vi "HFRR ADV v07.vi"() -> ()   [LabVIEW 2025] (continued)
                    n2291 = local write "Start Time"(TRUE ("Start Time")) -> ()
                    n2292 = property on="Stroke 2" class="DigNum (strict)"("Visible"=FALSE) -> ()  [unwired: 2 in, 2 out]
                    n2293 = case shown="False" w2888 {
                      frame False {
                        n2294 = property on="Heater Button" class="Bool (strict)"("DisabledEnum"=T15."Enabled" ("Disabled")) -> ()  [unwired: 2 in, 2 out]
                        n2295 = property on="Humidity" class="Bool (strict)"("DisabledEnum"=T15."Enabled" ("Disabled")) -> ()  [unwired: 2 in, 2 out]
                      }
                      frame True {
                      }
                    }
                    n2296 = case shown="False" "TestCompFlg" {
                      frame False {
                        n2297 = local read "StartFlg"() -> (w2896:bool)
                        n2298 = case shown="True" w2896 {
                          frame False {
                          }
                          frame True {
                            n2299 = flat-sequence {
                              frame #0 {
                                n2300 = local read "EVENT LOG"() -> (w2898:string)
                                n2301 = call "Event Log.vi"("Content"="Test was interrupted", "EVENT LOG"=w2898) -> ("EVENT LOG"=w2899:string)  [unwired: 8 in, 1 out]
                                n2302 = local write "EVENT LOG"(w2899) -> ()
                              }
                              frame #1 {
                                w2900 = FALSE ("StartFlg")
                                n2303 = local write "Heater Button"(w2900) -> ()
                                n2304 = local write "StartFlg"(w2900) -> ()
                                n2305 = local write "Humidity"(w2900) -> ()
                              }
                            }
                          }
                        }
                      }
                      frame True {
                      }
                    }
                    n2306 = local write "String 14"("Test will autostart once parameters reach the set value." ("String 14")) -> ()
                  }
                  frame True {
                    (unwired) FALSE ("Visible")
                    n2307 = property on="Stroke 2" class="DigNum (strict)"("Visible"=TRUE) -> ()  [unwired: 2 in, 2 out]
                    n2308 = property on="STOP 2" class="Bool (strict)"("Disabled"=u8 2) -> ()  [unwired: 2 in, 2 out]
                    n2309 = local write "String 14"(" Running....." ("String 14")) -> ()
                    n2310 = property on="Heater Button" class="Bool (strict)"("DisabledEnum"=T15."Disabled and Grayed Out" ("Disabled")) -> ()  [unwired: 2 in, 2 out]
                    n2311 = property on="Humidity" class="Bool (strict)"("DisabledEnum"=T15."Disabled and Grayed Out" ("Disabled")) -> ()  [unwired: 2 in, 2 out]
                    n2312 = case shown="True" "Start Time" {
                      selector: "Start Time" -> [_ w2914]
                      frame False {
                      }
                      frame True {
                        n2313 = Not(x=w2914) -> (.not. x?=w2913:bool)
                        n2314 = local write "Start Time"(w2913) -> ()
                        n2315 = local read "EVENT LOG"() -> (w2915:string)
                        n2316 = call "Event Log.vi"("Content"="Test in progress", "EVENT LOG"=w2915) -> ("EVENT LOG"=w2917:string)  [unwired: 8 in, 1 out]
                        n2317 = local write "EVENT LOG"(w2917) -> ()
                      }
                    }
                    n2318 = local read "Set Hz"() -> (w2911:dbl)
                    n2319 = call <vilib>:"Uniform White Noise Waveform.vi"() -> ("signal out"=w2910:waveform(dbl))  [unwired: 10 in, 1 out]
                    n2320 = Add(x=w2911, y=w2910) -> (x+y=w2909:waveform(dbl))
                    n2321 = Multiply(x=w2909, y=ext 0.1) -> (x*y=w2901:waveform(ext))
                    "StartFlg" <- TRUE ("StartFlg")
                  }
                }
                n2322 = case shown="True" w2878 {
                  frame False {
                  }
                  frame True {
                    n2323 = local write "clk"(10.0 ("clk")) -> ()
                    n2324 = Get Date/Time In Seconds() -> (seconds since 1Jan1904=w2920:timestamp)
                    n2325 = To Double Precision Float(number=w2920) -> (double precision float=w2918:dbl)
                    n2326 = local write "acq timer"(w2918) -> ()
                    n2327 = local write "act save time"(w2918) -> ()
                  }
                }
                n2328 = call "Elapsed Time"("Time Target (s)"="Countdown", "Reset"=w2867) -> ("Elapsed Time (s)"=w2872:dbl, "Time has Elapsed"=w2870:bool)  [unwired: 10 in, 6 out]
                "Countdown 2" <- w2872
                n2329 = Subtract(x=w2872, y=2.0) -> (x-y=w2875:dbl)
                n2330 = Less?(x=w2875, y="Countdown") -> (x < y?=w2873:bool)
                n2331 = And(x=w2873, y=w2870) -> (x .and. y?=w2869:bool)
                n2332 = case shown="True" w2869 {
                  frame False {
                  }
                  frame True {
                    (unwired) dbl[] [] ("History Data")
                    n2333 = local write "Engage"(FALSE ("Engage")) -> ()
                    n2334 = local write "RUN"(TRUE ("RUN")) -> ()
                    n2335 = local read "Humidity ( %RH )"() -> (→"Rh Before":dbl)
                  }
                }
                n2336 = local read "Test \nStatus"() -> (w2865:bool)
                n2337 = Multiply(x=w2859, y=10.0) -> (x*y=w2860:dbl)
                n2338 = Select(t=w2860, s=w2865, f=0.0) -> (s? t:f=w2864:dbl)
                n2339 = local write "Frequency ( Hz )"(w2864) -> ()
              }
              frame #1 {
                w2943 = 1000000.0 ("x")
                # "Elapsed time\ncof\nstroke\nAir temp\nTemp\nHumidity"
                # "acq timer\n\nact save time"
                # "convert to microseconds"
                n2340 = local read "COUNT"() -> (w2926:i32)
                n2341 = local read "Rate"() -> (w2939:dbl)
                n2342 = Divide(x=w2943, y=w2939) -> (x/y=w2944:dbl)
                n2343 = Greater Or Equal?(x=w2926, y=250) -> (x >= y?=w2925:bool)
                n2344 = Get Date/Time In Seconds() -> (seconds since 1Jan1904=w2946:timestamp)
                n2345 = case shown="True" w2925 {
                  frame False {
                    n2346 = local read "COUNT"() -> (w2947:i32)
                    n2347 = Increment(x=w2947) -> (x+1=w2948:i32)
                    n2348 = local write "COUNT"(w2948) -> ()
                  }
                  frame True {
                    n2349 = local write "COUNT"(0 ("COUNT")) -> ()
                  }
                }
                n2350 = local read "Samplingtime 2"() -> (w2924:dbl)
                n2351 = local read "act save time"() -> (w2941:dbl)
                n2352 = Divide(x=w2944, y=w2943) -> (x/y=w2942:dbl)
                n2353 = To Double Precision Float(number=w2946) -> (double precision float=w2935:dbl)
                n2354 = Add(x=w2941, y=w2924) -> (x+y=w2940:dbl)
                n2355 = local read "acq timer"() -> (w2945:dbl)
                n2356 = local read "COUNT"() -> (w2928:i32)
                n2357 = Greater Or Equal?(x=w2935, y=w2940) -> (x >= y?=w2923:bool)
                n2358 = Multiply(x=w2942, y=w2928) -> (x*y=w2934:dbl)
                n2359 = Subtract(x=w2935, y=w2945) -> (x-y=w2937:dbl)
                n2360 = local read "Save"() -> (w2938:bool)
                n2361 = Add(x=w2937, y=w2934) -> (x+y=w2921:dbl)
                "Elapsed time 3" <- w2921
                n2362 = And(x=w2923, y=w2938) -> (x .and. y?=w2936:bool)
                n2363 = Divide(x=w2921, y=60.0) -> (x/y=w2932:dbl)
                n2364 = local read "Test \nStatus"() -> (w2922:bool)
                n2365 = local read "clk"() -> (w2929:dbl)
                n2366 = Equal?(x=w2929, y=10.0) -> (x = y?=w2931:bool)
                n2367 = case shown="True" w2936 {
                  tunnel: w2935 -> [_ w3052]
                  tunnel: [FALSE ("Boolean 2") TRUE ("Boolean 2")] -> _
                  frame False {
                  }
                  frame True {
                    w3006 = ";" ("Substring")
                    # "Pid out/\nFreq response value"
                    n2368 = local write "act save time"(w3052) -> ()
                    n2369 = local read "FILE"() -> (w3000:string)
                    n2370 = call "file check.vi"("file name in"=w3000) -> ("error out"=w3003:errorcluster, "file name out"=w2998:string)  [unwired: 9 in]
                    n2371 = call "FILE PATH CREATION.vi"("error in"=w3003, "FILE NAME :"=w2998) -> ("FILE OUT"=w3001:path)  [unwired: 8 in, 1 out]
                    n2372 = Concatenate Strings(w2998, ".dgf" ("Substring")) -> (w3002:string)
                    n2373 = local read "FF 2"() -> (→"Frictional Force ( N )" →"Frictional Force ( N )":dbl)
                    n2374 = Build Path(base path=w3001, name or relative path=w3002) -> (appended path=w2997:path)
                    n2375 = local read "COF 2"() -> (w3011:dbl)
                    "cof" <- w3011
                    "Coefficient of Friction" <- w3011
                    "COF 4" <- w3011
                    "Coefficient of Friction" <- w3011
                    n2376 = local read "TEMP"() -> (w3014:dbl)
                    "Temp" <- w3014
                    "Temperature ( Deg C )" <- w3014
                    n2377 = local read "Humidity ( %RH )"() -> (w3013:dbl)
                    "Humidity ( %RH )" <- w3013
                    "Humidity ( %RH )" <- w3013
                    n2378 = local read "Frequency ( Hz )"() -> (w3020:dbl)
                    n2379 = local read "Elapsed time"() -> (w3045:dbl)
                    n2380 = local read "AIR TEMP"() -> (w3018:dbl)
                    n2381 = local read "PID-out"() -> (w3023:dbl)
                    n2382 = local write "Temperature ( Deg C )"(w3014) -> ()
                    n2383 = Number To Fractional String(number="measured_stroke", width (-)=i16 9 ("precision (6)"), precision (6)=i16 6) -> (F-format string=w3038:string)  [unwired: 1 in]
                    n2384 = Number To Fractional String(number=w3018, width (-)=i16 9 ("precision (6)"), precision (6)=i16 3) -> (F-format string=w3037:string)  [unwired: 1 in]
                    n2385 = Number To Fractional String(number=w3014, width (-)=i16 9 ("precision (6)"), precision (6)=i16 3) -> (F-format string=w3034:string)  [unwired: 1 in]
                    n2386 = Number To Fractional String(number=w3013, width (-)=i16 9 ("precision (6)"), precision (6)=i16 3) -> (F-format string=w3031:string)  [unwired: 1 in]
                    n2387 = Number To Fractional String(number=0.0, width (-)=i16 9 ("precision (6)"), precision (6)=i16 3) -> (F-format string=w3028:string)  [unwired: 1 in]
                    n2388 = Number To Fractional String(number=w3023, width (-)=i16 9 ("precision (6)"), precision (6)=i16 3) -> (F-format string=w3024:string)  [unwired: 1 in]
                    n2389 = Number To Fractional String(number=w3020, width (-)=i16 9 ("precision (6)"), precision (6)=i16 3) -> (F-format string=w3019:string)  [unwired: 1 in]
                    n2390 = Number To Fractional String(number=w3011, width (-)=i16 9 ("precision (6)"), precision (6)=i16 6) -> (F-format string=w3046:string)  [unwired: 1 in]
                    n2391 = Number To Fractional String(number=w3045, width (-)=i16 14 ("precision (6)"), precision (6)=i16 3) -> (F-format string=w3047:string)  [unwired: 1 in]
                    n2392 = Bundle("y"=1.02, "measured_stroke"="measured_stroke", "y"=0.98) -> (w3012:cluster{"y":dbl, "measured_stroke":dbl, "y":dbl})  [unwired: 1 in]
                    n2393 = Number To Fractional String(number="Ambient Humidity :", width (-)=i16 9 ("precision (6)"), precision (6)=i16 6) -> (F-format string=w3004:string)  [unwired: 1 in]
                    n2394 = local read "RUN"() -> (w3010:bool)
                    n2395 = case shown="True" w3010 {
                      tunnel: w3012 -> [_ w3057]
                      tunnel: "measured_stroke" -> [_ w3056]
                      tunnel: "measured_stroke" -> [_ w3055]
                      tunnel: "measured_stroke" -> [_ w3054]
                      frame False {
                      }
                      frame True {
                        "Stroke ( mm )" <- w3057
                        "Stroke ( mm )" <- w3057
                        "Stroke 4" <- w3056
                        "Stroke 3" <- w3055
                        "Stroke 2" <- w3054
                      }
                    }
                    n2396 = Concatenate Strings(w3047, w3006, w3046, w3006, w3038, w3006, w3037, w3006, w3034, w3006, w3031, w3006, w3028, w3006, w3024, w3006, w3019, w3006, w3004, "\r") -> (w3044:string)
                    n2397 = call <vilib>:"Write Characters To File.vi"("append to file? (new file:F)"=TRUE, "character string"=w3044, "file path (dialog if empty)"=w2997) -> ()  [unwired: 2 in, 1 out]
                    "refresh flag" <- TRUE ("refresh flag")
                  }
                }
                n2398 = case shown="True" w2922 {
                  tunnel: w2932 -> [_ w2958]
                  tunnel: w2937 -> [_ w2968]
                  tunnel: [0.0 w2964] -> _
                  tunnel: w2931 -> [_ w2963]
                  tunnel: [0.0 w2962] -> _
                  tunnel: w2921 -> [_ w2962]
                  tunnel: w2935 -> [w2951 _]
                  frame False {
                    n2399 = local write "acq timer"(w2951) -> ()
                    n2400 = local write "Test Duration Status"(0.0 ("Test Duration Status")) -> ()
                  }
                  frame True {
                    n2401 = local read "Set Hz"() -> (w2965:dbl)
                    n2402 = local write "Elapsed time"(w2958) -> ()
                    n2403 = local read "test time"() -> (w2957:dbl)
                    n2404 = Multiply(x=w2968, y=w2965) -> (x*y=w2967:dbl)
                    n2405 = case shown="False" w2963 {
                      tunnel: w2967 -> [w2969 _]
                      tunnel: [w2969 1.0] -> w2964
                      frame False {
                        n2406 = local write "Cycles elapsed"(w2969) -> ()
                      }
                      frame True {
                      }
                    }
                    n2407 = Greater?(x=w2958, y=w2957) -> (0:w2966:bool)
                    n2408 = Subtract(x=w2957, y=w2958) -> (x-y=w2956:dbl)
                    "time" <- w2956
                    n2409 = Multiply(x=w2956, y=60.0) -> (x*y=w2955:dbl)
                    n2410 = local write "Time Remaining"(w2955) -> ()
                    n2411 = local write "Remaining Time"(w2955) -> ()
                    n2412 = case shown="True" w2966 {
                      frame False {
                      }
                      frame True {
                        n2413 = stacked-sequence {
                          frame #0 {
                            w2974 = T15."Enabled" ("Disabled")
                            w2973 = FALSE ("TEST FILE NAM,E SAVED")
                            w2975 = "" ("FILE")
                            w2976 = TRUE ("Visible")
                            n2414 = local write "Humidity"(FALSE ("Humidity")) -> ()
                            n2415 = local write "RUN"(FALSE ("OK Button 2")) -> ()
                            n2416 = local write "Heater Button"(FALSE ("Heater Button")) -> ()
                            n2417 = local write "Auto Start Test"(FALSE ("Auto Start Test")) -> ()
                            n2418 = local write "TestCompFlg"(TRUE ("StpFlg")) -> ()
                            n2419 = local read "Humidity ( %RH )"() -> (→"Rh After":dbl)
                            n2420 = property on="STOP 2" class="Bool (strict)"("Disabled"=u8 0) -> ()  [unwired: 2 in, 2 out]
                            n2421 = local read "EVENT LOG"() -> (w2981:string)
                            n2422 = call "Event Log.vi"("Content"="Test Completed", "EVENT LOG"=w2981) -> ("EVENT LOG"=w2980:string)  [unwired: 8 in, 1 out]
                            n2423 = property on="RUN" class="Bool (strict)"("Visible"=w2976) -> ()  [unwired: 2 in, 2 out]
                            n2424 = property on="Auto Start Test" class="Bool (strict)"("Visible"=w2976) -> ()  [unwired: 2 in, 2 out]
                            n2425 = local write "Batch Ref Num :"(w2975) -> ()
                            n2426 = local write "FILE"(w2975) -> ()
                            n2427 = local write "EVENT LOG"(w2980) -> ()
                            n2428 = local write "TEST FILE NAM,E SAVED"(w2973) -> ()
                            n2429 = local write "Fuel Discription :"(w2975) -> ()
                            n2430 = local write "START TEMP"(w2973) -> ()
                            n2431 = local write "Remarks :"(w2975) -> ()
                            n2432 = local write "Main Dashboard Buttons"(T1."Imaging" ("Main Dashboard Buttons")) -> ()
                            n2433 = local write "Main Tab"(T2."Adv Scar" ("Main Tab")) -> ()
                            n2434 = property on="FRICVALZ 2" class="Bool (strict)"("DisabledEnum"=w2974) -> ()  [unwired: 2 in, 2 out]
                            n2435 = property on="FRICVALZ 3" class="Bool (strict)"("DisabledEnum"=w2974) -> ()  [unwired: 2 in, 2 out]
                            n2436 = property on="FRICVALZ 4" class="Bool (strict)"("DisabledEnum"=w2974) -> ()  [unwired: 2 in, 2 out]
                          }
                          frame #1 {
                            n2437 = Wait (ms)(milliseconds to wait=u32 1500) -> ()  [unwired: 1 out]
                          }
                          frame #2 {
                            n2438 = local write "Command"("VC;0") -> ()
                          }
                          frame #3 {
                            n2439 = Wait (ms)(milliseconds to wait=u32 1500) -> ()  [unwired: 1 out]
                          }
                          frame #4 {
                            n2440 = local write "Command"("ST;0") -> ()
                          }
                          frame #5 {
                            n2441 = Wait (ms)(milliseconds to wait=u32 1500) -> ()  [unwired: 1 out]
                          }
                          frame #6 {
                            n2442 = local write "Command"("HE;0" ("Command")) -> ()
                          }
                          frame #7 {
                            n2443 = Wait (ms)(milliseconds to wait=u32 1500) -> ()  [unwired: 1 out]
                          }
                        }
                      }
                    }
                    n2444 = Divide(x=w2958, y=w2957) -> (x/y=w2961:dbl)
                    n2445 = Multiply(x=w2961, y=100.0) -> (x*y=w2959:dbl)
                    n2446 = local write "Test Duration Status"(w2959) -> ()
                  }
                }
              }
              frame #2 {
                n2447 = case shown="True" "Heater Button" {
                  tunnel: [0.0 ("output") w3067] -> w3058
                  frame False {
                    w3061 = TRUE ("tmpchk")
                    n2448 = local read "TEMP"() -> (w3062:dbl)
                    n2449 = local write "Reset 4"(w3061) -> ()
                    n2450 = local write "Temp ini"(w3062) -> ()
                    n2451 = local write "tmpchk"(w3061) -> ()
                    n2452 = local write "reinit"(TRUE ("reinit")) -> ()
                    n2453 = local write "manual temp log"(TRUE ("manual temp log")) -> ()
                  }
                  frame True {
                    n2454 = local read "Auto Start Test"() -> (w3066:bool)
                    n2455 = case shown="True" FALSE {
                      tunnel: [_ w3082] -> w3067
                      frame False {
                      }
                      frame True {
                        # "Logic to turn off\nthe heater when \ntemp is not rising.\nTime - 60 sec\nDelta t- 5°c"
                        n2456 = local read "Temp ini"() -> (w3071:dbl)
                        n2457 = Less?(x=w3071, y=53.0) -> (x < y?=w3069:bool)
                        n2458 = And(x="tmpchk", y=w3069) -> (x .and. y?=w3072:bool)
                        n2459 = case shown="True" w3072 {
                          frame False {
                          }
                          frame True {
                            n2460 = call "Elapsed Time8"("Time Target (s)"=300.0, "Reset"="Reset 4") -> ("Time has Elapsed"=w3085:bool)  [unwired: 10 in, 7 out]
                            n2461 = flat-sequence {
                              tunnel: w3085 -> [_]
                              frame #0 {
                                n2462 = local write "Reset 4"(FALSE ("Reset 4")) -> ()
                              }
                            }
                            n2463 = case shown="True" w3085 {
                              frame False {
                              }
                              frame True {
                                n2464 = local read "Temp ini"() -> (w3092:dbl)
                                n2465 = Add(x=w3092, y=5.0) -> (x+y=w3090:dbl)
                                n2466 = local read "TEMP"() -> (w3093:dbl)
                                n2467 = Greater?(x=w3093, y=w3090) -> (0:w3091:bool)
                                n2468 = case shown="False" w3091 {
                                frame False {
                                n2469 = local write "Heater Button"(FALSE ("Heater Button")) -> ()
                                }
                                frame True {
                                n2470 = local write "tmpchk"(FALSE ("tmpchk")) -> ()
                                }
                                }
                              }
                            }
                          }
                        }
                        n2471 = local read "Set Temp"() -> (w3080:dbl)
                        n2472 = local read "TEMP"() -> (w3074:dbl)
                        n2473 = call-poly <vilib>:"PID.vi"("reinitialize? (F)"="reinit", "dt (s)"=-1.0, "process variable"=w3074, "setpoint"=w3080) -> ("output"=w3077:dbl)  [unwired: 6 in, 1 out]
                        n2474 = Subtract(x=w3080, y=w3074) -> (x-y=w3081:dbl)
                        n2475 = Add(x=w3080, y=0.5) -> (x+y=w3078:dbl)
                        n2476 = Greater Or Equal?(x=w3074, y=w3078) -> ()  [unwired: 1 out]
                        n2477 = Select(t=0.0, s=FALSE, f=w3077) -> (s? t:f=w3076:dbl)
                        "PID output" <- w3076
                        n2478 = flat-sequence {
                          tunnel: w3076 -> [w3096]
                          tunnel: [w3096] -> w3082
                          frame #0 {
                            n2479 = local write "reinit"(FALSE ("reinit")) -> ()
                          }
                        }
                        n2480 = Bundle(w3081, "output"=w3076, "TEMP"=w3074) -> ()  [unwired: 1 in, 1 out]
                      }
                    }
                    n2481 = case shown="False" w3066 {
                      frame False {
                        n2482 = local read "Set Temp"() -> (w3104:dbl)
                        n2483 = local read "TEMP"() -> (w3103:dbl)
                        n2484 = Subtract(x=w3104, y=w3103) -> (x-y=w3102:dbl)
                        n2485 = Absolute Value(x=w3102) -> (abs(x)=w3101:dbl)
                        n2486 = Less?(x=w3101, y=0.5) -> (x < y?=w3099:bool)
                        n2487 = case shown="True" w3099 {
                          tunnel: "manual temp log" -> [_ w3105]
                          frame False {
                          }
                          frame True {
                            n2488 = case shown="True" w3105 {
                              selector: w3105 -> [_ w3106]
                              frame False {
                              }
                              frame True {
                                # "#Event log"
                                n2489 = Not(x=w3106) -> (.not. x?=w3107:bool)
                                n2490 = local write "manual temp log"(w3107) -> ()
                                n2491 = local read "EVENT LOG"() -> (w3110:string)
                                n2492 = call "Event Log.vi"("Content"="Target Temperature reached", "EVENT LOG"=w3110) -> ("EVENT LOG"=w3109:string)  [unwired: 8 in, 1 out]
                                n2493 = local write "EVENT LOG"(w3109) -> ()
                              }
                            }
                          }
                        }
                      }
                      frame True {
                        n2494 = local write "manual temp log"(TRUE ("manual temp log")) -> ()
                      }
                    }
                  }
                }
                "PID-out" <- w3058
              }
              frame #3 {
                n2495 = local read "TEMP"() -> (w3112:dbl)
                n2496 = Greater Or Equal?(x=w3112, y="Set Temp 2") -> (x >= y?=w3117:bool)
                n2497 = case shown="True" w3117 {
                  tunnel: [FALSE TRUE] -> w3115
                  frame False {
                  }
                  frame True {
                  }
                }
                "Status 13" <- w3115
                n2498 = And(x=w3115, y="trip1 8") -> (x .and. y?=w3114:bool)
                n2499 = case shown="True" w3114 {
                  frame False {
                    n2500 = local write "Heater Trip Temp"(TRUE ("Heater Trip Temp")) -> ()
                  }
                  frame True {
                    w3120 = FALSE ("OK Button 2")
                    n2501 = case shown="True" "Heater Trip Temp" {
                      selector: "Heater Trip Temp" -> [_ w3122]
                      frame False {
                      }
                      frame True {
                        n2502 = Not(x=w3122) -> (.not. x?=w3121:bool)
                        n2503 = local read "EVENT LOG"() -> (w3125:string)
                        n2504 = local write "Heater Trip Temp"(w3121) -> ()
                        n2505 = call "Event Log.vi"("Content"="Heater Trip", "EVENT LOG"=w3125) -> ("EVENT LOG"=w3124:string)  [unwired: 8 in, 1 out]
                        n2506 = local write "EVENT LOG"(w3124) -> ()
                      }
                    }
                    n2507 = local write "RUN"(w3120) -> ()
                    n2508 = property on="Auto Start Test" class="Bool (strict)"("Value"=w3120) -> ()  [unwired: 2 in, 2 out]
                    n2509 = local write "Heater Button"(w3120) -> ()
                  }
                }
              }
            }
            n2510 = case shown="False" w2856 {
              frame False {
                n2511 = disable-structure shown="Enabled" {
                  frame Disabled {
                    n2512 = stacked-sequence {
                      frame #0 {
                        n2513 = local write "RUN"(FALSE ("OK Button 2")) -> ()
                      }
                      frame #1 {
                      }
                    }
                  }
                  frame Enabled {
                  }
                }
              }
              frame True {
              }
            }
          }
        }
        n2514 = case shown="True" w2659 {
          frame False {
            n2515 = local read "Rt 3"() -> (w2787:bool)
            n2516 = case shown="True" w2787 {
              frame False {
              }
              frame True {
                n2517 = local write "Json End Flg"(TRUE ("Upld AR 2")) -> ()
                n2518 = local write "Rt 3"(FALSE ("Rt 3")) -> ()
              }
            }
            "Rt" <- TRUE ("Rt")
            "Rt 2" <- FALSE ("Rt")
          }
          frame True {
            n2519 = local read "Rt"() -> (w2794:bool)
            n2520 = local write "Rt 2"(TRUE ("Rt 2")) -> ()
            n2521 = case shown="True" w2794 {
              frame False {
              }
              frame True {
                w2795 = TRUE ("Upld AR 2")
                n2522 = local write "Rt"(FALSE ("Rt")) -> ()
                n2523 = local write "Upld AR"(w2795) -> ()
                n2524 = local write "Json St Flg"(w2795) -> ()
              }
            }
            "Rt 3" <- TRUE ("Rt 3")
          }
        }
        n2525 = case shown="True" w2660 {
          frame False {
            n2526 = local write "tfalg"(0.0 ("tfalg")) -> ()
          }
          frame True {
            n2527 = local read "tfalg"() -> (w2805:dbl)
            n2528 = Equal?(x=w2805, y=0.0) -> (x = y?=w2806:bool)
            n2529 = case shown="True" w2806 {
              frame False {
              }
              frame True {
                n2530 = local read "Total No. of Tests"() -> (w2809:dbl)
                n2531 = local write "tfalg"(1.0 ("tfalg")) -> ()
                n2532 = local write "acq 2"(FALSE ("acq 2")) -> ()
                n2533 = Wait (ms)(milliseconds to wait=u32 200) -> ()  [unwired: 1 out]
                n2534 = Increment(x=w2809) -> (x+1=w2808:dbl)
                n2535 = local write "Total No. of Tests"(w2808) -> ()
              }
            }
          }
        }
        n2536 = local read "airtempflg"() -> (w2648:bool)
        n2537 = Or(x=w2648, y=w2646) -> (x .or. y?=w2649:bool)
        n2538 = Insert Into Array(array=string[] ["Air Temperature has reached set value,", "Humidity has reached set value,", "Sample Temperaturehas reached set value,", ""], index=0, new element="") -> (w2634:string[])
        n2539 = Build Array(w2639, w2638, w2637) -> (w2635:i32[])
        n2540 = for {
          tunnel: w2635 -> [w2777] mode=indexing
          tunnel: w2634 -> [w2776]
          shift-right: [w2773] -> w2633
          shift-left: "" -> [w2775]
          n2541 = Index Array(array=w2776, index=w2777) -> (element=w2774:string)
          n2542 = Concatenate Strings(w2774, w2775) -> (w2773:string)
        }
        n2543 = disable-structure shown="Disabled" {
          disable-tunnel: w2649 -> [w2726 _]
          disable-tunnel: w2644 -> [w2725 _]
          disable-tunnel: w2642 -> [w2724 _]
          frame Disabled {
            n2544 = Compound Arithmetic op=AND(w2726, w2725, w2724) -> ()  [unwired: 1 out]
            n2545 = case shown="True" {
              selector: _ -> [_ _]
              frame False {
              }
              frame True {
                w2727 = FALSE ("autostrtflg")
                n2546 = local write "RUN"(TRUE ("RUN")) -> ()
                n2547 = local write "autostart"(w2727) -> ()
                n2548 = local write "autostrtflg"(w2727) -> ()
                n2549 = local write "String 14"(" Running....." ("String 14")) -> ()
              }
            }
          }
          frame Enabled {
          }
        }
        n2550 = local write "autostart 2"(w2633) -> ()
        n2551 = local read "Reset Graph"() -> (w2622:bool)
        n2552 = case shown="True" "Save & Continue" {
          frame False {
          }
          frame True {
            n2553 = while {
              tunnel: "0123456789abcdefghijklmnopqrstuvwxyzABCDEFGHIJKLMNOPQRSTUVWXYZ" ("string 2") -> [w2821]
              shift-right: [w2819] -> w2814
              shift-left: "" -> [w2818]
              i -> [w2828]
              stop <- w2827 stop-if-true
              n2554 = Random Number (0-1)() -> (number: 0 to 1=w2822:dbl)
              n2555 = Multiply(x=w2822, y=62.0) -> (x*y=w2824:dbl)
              n2556 = Decrement(x="Length") -> (x-1=w2817:i16)
              n2557 = To Word Integer(number=w2824) -> (16bit integer=w2825:i16)
              n2558 = String Subset(string=w2821, offset (0)=w2825, length (rest)=1 ("length (rest)")) -> (substring=w2820:string)
              n2559 = Greater Or Equal?(x=w2828, y=w2817) -> (x >= y?=w2827:bool)
              n2560 = Concatenate Strings(w2820, w2818) -> (w2819:string)
            }
            n2561 = local write "UUID"(w2814) -> ()
          }
        }
        n2562 = case shown="True" w2622 {
          selector: w2622 -> [_ w2676]
          frame False {
          }
          frame True {
            w2690 = 0.0 ("X Scale.Range:Maximum")
            n2563 = Not(x=w2676) -> (.not. x?=w2675:bool)
            n2564 = local write "Reset Graph"(w2675) -> ()
            n2565 = property on="Electrical Contact Resistance ( % )" class="WFChart (strict)"("XScale.Maximum"=600.0 ("X Scale.Range:Maximum"), "XScale.Minimum"=0.0 ("X Scale.Range:Minimum"), "YScale.Maximum"=100.0 ("Y Scale.Range:Maximum"), "YScale.Minimum"=0.0 ("Y Scale.Range:Minimum")) -> ()  [unwired: 2 in, 2 out]
            n2566 = property on="Frictional Force ( N )" class="WFChart (strict)"("XScale.Maximum"=600.0 ("X Scale.Range:Maximum"), "XScale.Minimum"=0.0 ("X Scale.Range:Minimum"), "YScale.Maximum"=100.0 ("Y Scale.Range:Maximum"), "YScale.Minimum"=0.0 ("Y Scale.Range:Minimum")) -> ()  [unwired: 2 in, 2 out]
            n2567 = property on="Temperature ( Deg C )" class="WFChart (strict)"("XScale.Maximum"=600.0 ("X Scale.Range:Maximum"), "XScale.Minimum"=0.0 ("X Scale.Range:Minimum"), "YScale.Maximum"=100.0 ("Y Scale.Range:Maximum"), "YScale.Minimum"=0.0 ("Y Scale.Range:Minimum")) -> ()  [unwired: 2 in, 2 out]
            n2568 = property on="Humidity ( %RH )" class="WFChart (strict)"("XScale.Maximum"=600.0 ("X Scale.Range:Maximum"), "XScale.Minimum"=0.0 ("X Scale.Range:Minimum"), "YScale.Maximum"=100.0 ("Y Scale.Range:Maximum"), "YScale.Minimum"=0.0 ("Y Scale.Range:Minimum")) -> ()  [unwired: 2 in, 2 out]
            n2569 = property on="Coefficient of Friction" class="WFChart (strict)"("XScale.Maximum"=600.0 ("X Scale.Range:Maximum"), "XScale.Minimum"=0.0 ("X Scale.Range:Minimum"), "YScale.Maximum"=100.0 ("Y Scale.Range:Maximum"), "YScale.Minimum"=0.0 ("Y Scale.Range:Minimum")) -> ()  [unwired: 2 in, 2 out]
            n2570 = property on="Stroke ( mm )" class="WFChart (strict)"("XScale.Maximum"=600.0 ("X Scale.Range:Maximum"), "XScale.Minimum"=0.0 ("X Scale.Range:Minimum"), "YScale.Maximum"=100.0 ("Y Scale.Range:Maximum"), "YScale.Minimum"=0.0 ("Y Scale.Range:Minimum")) -> ()  [unwired: 2 in, 2 out]
            n2571 = property on="Electrical Contact Resistance ( % )" class="WFChart (strict)"("XScale.Minimum"=0.0 ("X Scale.Range:Minimum"), "XScale.Maximum"=600.0 ("X Scale.Range:Maximum"), "YScale.Minimum"=0.0 ("Y Scale.Range:Minimum"), "YScale.Maximum"=100.0 ("Y Scale.Range:Maximum")) -> ()  [unwired: 2 in, 2 out]
            n2572 = property on="Temperature ( Deg C )" class="WFChart (strict)"("XScale.Minimum"=0.0 ("X Scale.Range:Minimum"), "XScale.Maximum"=600.0 ("X Scale.Range:Maximum"), "YScale.Minimum"=0.0 ("Y Scale.Range:Minimum"), "YScale.Maximum"=100.0 ("Y Scale.Range:Maximum")) -> ()  [unwired: 2 in, 2 out]
            n2573 = property on="Coefficient of Friction" class="WFChart (strict)"("XScale.Minimum"=0.0 ("X Scale.Range:Minimum"), "XScale.Maximum"=600.0 ("X Scale.Range:Maximum"), "YScale.Maximum"=1.0 ("X Scale.Range:Minimum"), "YScale.Minimum"=0.0 ("X Scale.Range:Minimum")) -> ()  [unwired: 2 in, 2 out]
            n2574 = property on="Frictional Force ( N )" class="WFChart (strict)"("XScale.Maximum"=600.0 ("X Scale.Range:Maximum"), "XScale.Minimum"=w2690, "YScale.Maximum"=10.0 ("Y Scale.Range:Maximum"), "YScale.Minimum"=w2690) -> ()  [unwired: 2 in, 2 out]
            n2575 = property on="Stroke ( mm )" class="WFChart (strict)"("XScale.Maximum"=600.0 ("X Scale.Range:Maximum"), "XScale.Minimum"=0.0 ("X Scale.Range:Minimum"), "YScale.Maximum"=100.0 ("Y Scale.Range:Maximum"), "YScale.Minimum"=0.0 ("Y Scale.Range:Minimum")) -> ()  [unwired: 2 in, 2 out]
            n2576 = property on="Humidity ( %RH )" class="WFChart (strict)"("XScale.Maximum"=600.0 ("X Scale.Range:Maximum"), "XScale.Minimum"=0.0 ("X Scale.Range:Minimum"), "YScale.Maximum"=100.0 ("Y Scale.Range:Maximum"), "YScale.Minimum"=0.0 ("Y Scale.Range:Minimum")) -> ()  [unwired: 2 in, 2 out]
          }
        }
      }
      frame "Compare Files" {
        # "Elapsed time\ncof\nstroke\nAir temp\nTemp\nHumidity"
        n2577 = case shown="True" "RST CP 3" {
          frame False {
          }
          frame True {
            n2578 = property on="Air Temp ( °C ) vs Humidity ( % RH )" class="XYGraph (strict)"("X Scale.Range:Minimum"=18.0, "X Scale.Range:Maximum"=28.0 ("X Scale.Range:Minimum"), "Y Scale.Range:Minimum"=30.0 ("X Scale.Range:Minimum"), "Y Scale.Range:Maximum"=70.0 ("X Scale.Range:Minimum")) -> ()  [unwired: 2 in, 2 out]
          }
        }
        n2579 = case shown="True" "RST CP 2" {
          frame False {
          }
          frame True {
            n2580 = property on="XY Graph 13" class="XYGraph (strict)"("Y Scale.Display Format:Precision"=u8 0 ("Y Scale.Format & Precision:Precision")) -> ()  [unwired: 2 in, 2 out]
            n2581 = property on="XY Graph 13" class="XYGraph (strict)"("X Scale.Range:Minimum"=0.0, "X Scale.Range:Maximum"=75.0, "Y Scale.Range:Minimum"=0.0, "Y Scale.Range:Maximum"=100.0) -> ()  [unwired: 2 in, 2 out]
          }
        }
        n2582 = case shown="True" "RSTV1 2" {
          frame False {
          }
          frame True {
            n2583 = property on="Humidity ( %RH )" class="XYGraph (strict)"("Y Scale.Display Format:Precision"=u8 0 ("Y Scale.Format & Precision:Precision")) -> ()  [unwired: 2 in, 2 out]
            n2584 = property on="Humidity ( %RH )" class="XYGraph (strict)"("X Scale.Range:Minimum"=0.0, "X Scale.Range:Maximum"=75.0, "Y Scale.Range:Minimum"=48.0, "Y Scale.Range:Maximum"=58.0) -> ()  [unwired: 2 in, 2 out]
          }
        }
        n2585 = case shown="True" "RST CP" {
          frame False {
          }
          frame True {
            n2586 = property on="Sample Temperature ( °C )" class="XYGraph (strict)"("Y Scale.Display Format:Precision"=u8 2 ("Y Scale.Format & Precision:Precision")) -> ()  [unwired: 2 in, 2 out]
            n2587 = property on="Sample Temperature ( °C )" class="XYGraph (strict)"("X Scale.Range:Minimum"=0.0, "X Scale.Range:Maximum"=75.0, "Y Scale.Range:Minimum"=58.0, "Y Scale.Range:Maximum"=62.0) -> ()  [unwired: 2 in, 2 out]
          }
        }
        n2588 = case shown="True" "RSTV1 3" {
          frame False {
          }
          frame True {
            n2589 = property on="Air Temperature  ( °C )" class="XYGraph (strict)"("Y Scale.Display Format:Precision"=u8 2 ("Y Scale.Format & Precision:Precision")) -> ()  [unwired: 2 in, 2 out]
            n2590 = property on="Air Temperature  ( °C )" class="XYGraph (strict)"("X Scale.Range:Minimum"=0.0 ("Y Scale.Range:Minimum"), "X Scale.Range:Maximum"=75.0 ("Y Scale.Range:Maximum"), "Y Scale.Range:Minimum"=20.0 ("X Scale.Range:Minimum"), "Y Scale.Range:Maximum"=26.0 ("X Scale.Range:Maximum")) -> ()  [unwired: 2 in, 2 out]
          }
        }
        n2591 = case shown="True" "rstv2" {
          frame False {
          }
          frame True {
            n2592 = property on="Coefficient Of Friction" class="XYGraph (strict)"("Y Scale.Display Format:Precision"=u8 3 ("Y Scale.Format & Precision:Precision")) -> ()  [unwired: 2 in, 2 out]
            n2593 = property on="Coefficient Of Friction" class="XYGraph (strict)"("X Scale.Range:Minimum"=0.0 ("Y Scale.Range:Maximum"), "X Scale.Range:Maximum"=75.0, "Y Scale.Range:Minimum"=0.0, "Y Scale.Range:Maximum"=1.0 ("X Scale.Range:Minimum")) -> ()  [unwired: 2 in, 2 out]
          }
        }
        n2594 = case shown="True" "RSTV1 4" {
          frame False {
          }
          frame True {
            n2595 = property on="Stroke ( mm )" class="XYGraph (strict)"("Y Scale.Display Format:Precision"=u8 2 ("Y Scale.Format & Precision:Precision")) -> ()  [unwired: 2 in, 2 out]
            n2596 = property on="Stroke ( mm )" class="XYGraph (strict)"("X Scale.Range:Minimum"=0.0 ("Y Scale.Range:Maximum"), "X Scale.Range:Maximum"=75.0 ("X Scale.Range:Minimum"), "Y Scale.Range:Minimum"=0.98, "Y Scale.Range:Maximum"=1.02) -> ()  [unwired: 2 in, 2 out]
          }
        }
        n2597 = case shown="True" "OPEN 1" {
          frame False {
          }
          frame True {
            (unwired) 0  # existing file
            w3401 = "Choose a datalog file to open"  # prompt
            n2598 = local write "OPEN 1"(FALSE ("OPEN 1")) -> ()
            n2599 = String To Path(string="C:\\LAB-IQ\\Data\\") -> (path=w3386:path)
            n2600 = File Dialog(6:"*.dgf" ("pattern"), 7:w3401, 11:w3386) -> (0:w3384:errorcluster, 3:w3392:path)  [unwired: 4 in, 2 out]
            n2601 = Unbundle(w3384) -> ()  [unwired: 3 out]
            n2602 = Strip Path(path=w3392) -> (name=w3391:string)  [unwired: 1 out]
            n2603 = Path To String(path=w3392) -> (string=w3387:string)
            "string1" <- w3387
            n2604 = Match Pattern(string=w3391, regular expression=".dgf") -> (before substring=→"String Control":string)  [unwired: 1 in, 3 out]
            n2605 = Match Pattern(string=w3387, regular expression=".dgf" ("substring (\"\")")) -> (before substring=w3397:string)  [unwired: 1 in, 3 out]
            n2606 = Concatenate Strings(w3397, ".duf" ("Substring")) -> (w3393:string)
            n2607 = String To Path(string=w3393) -> (path=w3398:path)
            n2608 = call <vilib>:"Read Characters From File.vi"("file path (dialog if empty)"=w3398, "start of read offset (chars.:0)"=60 ("start of read offset (chars.: 0)")) -> ("character string"=→"String Control 2":string)  [unwired: 4 in, 3 out]
          }
        }
        n2609 = case shown="True" "OPEN 2" {
          frame False {
          }
          frame True {
            (unwired) 0  # existing file
            w3419 = "Choose a datalog file to open"  # prompt
            n2610 = local write "OPEN 2"(FALSE ("OPEN 1")) -> ()
            n2611 = String To Path(string="C:\\LAB-IQ\\Data\\") -> (path=w3404:path)
            n2612 = File Dialog(6:"*.dgf" ("pattern"), 7:w3419, 11:w3404) -> (0:w3402:errorcluster, 3:w3410:path)  [unwired: 4 in, 2 out]
            n2613 = Unbundle(w3402) -> ()  [unwired: 3 out]
            n2614 = Strip Path(path=w3410) -> (name=w3408:string)  [unwired: 1 out]
            n2615 = Path To String(path=w3410) -> (string=w3405:string)
            "string1 2" <- w3405
            n2616 = Match Pattern(string=w3408, regular expression=".dgf") -> (before substring=→"String Control 3":string)  [unwired: 1 in, 3 out]
            n2617 = Match Pattern(string=w3405, regular expression=".dgf" ("substring (\"\")")) -> (before substring=w3416:string)  [unwired: 1 in, 3 out]
            n2618 = Concatenate Strings(w3416, ".duf" ("Substring")) -> (w3413:string)
            n2619 = String To Path(string=w3413) -> (path=w3411:path)
            n2620 = call <vilib>:"Read Characters From File.vi"("file path (dialog if empty)"=w3411, "start of read offset (chars.:0)"=60 ("start of read offset (chars.: 0)")) -> ("character string"=→"String Control 4":string)  [unwired: 4 in, 3 out]
          }
        }
        n2621 = case shown="True" "OPEN 3" {
          frame False {
          }
          frame True {
            (unwired) 0  # existing file
            w3437 = "Choose a datalog file to open"  # prompt
            n2622 = local write "OPEN 3"(FALSE ("OPEN 1")) -> ()
            n2623 = String To Path(string="C:\\LAB-IQ\\Data\\") -> (path=w3422:path)
            n2624 = File Dialog(6:"*.dgf" ("pattern"), 7:w3437, 11:w3422) -> (0:w3420:errorcluster, 3:w3428:path)  [unwired: 4 in, 2 out]
            n2625 = Unbundle(w3420) -> ()  [unwired: 3 out]
            n2626 = Strip Path(path=w3428) -> (name=w3426:string)  [unwired: 1 out]
            n2627 = Path To String(path=w3428) -> (string=w3423:string)
            "string1 3" <- w3423
            n2628 = Match Pattern(string=w3426, regular expression=".dgf") -> (before substring=→"String Control 5":string)  [unwired: 1 in, 3 out]
            n2629 = Match Pattern(string=w3423, regular expression=".dgf" ("substring (\"\")")) -> (before substring=w3433:string)  [unwired: 1 in, 3 out]
            n2630 = Concatenate Strings(w3433, ".duf" ("Substring")) -> (w3430:string)
            n2631 = String To Path(string=w3430) -> (path=w3434:path)
            n2632 = call <vilib>:"Read Characters From File.vi"("file path (dialog if empty)"=w3434, "start of read offset (chars.:0)"=60 ("start of read offset (chars.: 0)")) -> ("character string"=→"String Control 6":string)  [unwired: 4 in, 3 out]
          }
        }
        n2633 = case shown="True" "OPEN 4" {
          frame False {
          }
          frame True {
            (unwired) 0  # existing file
            w3455 = "Choose a datalog file to open"  # prompt
            n2634 = local write "OPEN 4"(FALSE ("OPEN 1")) -> ()
            n2635 = String To Path(string="C:\\LAB-IQ\\Data\\") -> (path=w3440:path)
            n2636 = File Dialog(6:"*.dgf" ("pattern"), 7:w3455, 11:w3440) -> (0:w3438:errorcluster, 3:w3446:path)  [unwired: 4 in, 2 out]
            n2637 = Unbundle(w3438) -> ()  [unwired: 3 out]
            n2638 = Strip Path(path=w3446) -> (name=w3444:string)  [unwired: 1 out]
            n2639 = Path To String(path=w3446) -> (string=w3441:string)
            "string1 4" <- w3441
            n2640 = Match Pattern(string=w3444, regular expression=".dgf") -> (before substring=→"String Control 7":string)  [unwired: 1 in, 3 out]
            n2641 = Match Pattern(string=w3441, regular expression=".dgf" ("substring (\"\")")) -> (before substring=w3451:string)  [unwired: 1 in, 3 out]
            n2642 = Concatenate Strings(w3451, ".duf" ("Substring")) -> (w3448:string)
            n2643 = String To Path(string=w3448) -> (path=w3452:path)
            n2644 = call <vilib>:"Read Characters From File.vi"("file path (dialog if empty)"=w3452, "start of read offset (chars.:0)"=60 ("start of read offset (chars.: 0)")) -> ("character string"=→"String Control 8":string)  [unwired: 4 in, 3 out]
          }
        }
      }
      frame "About" {
        # "Elapsed time\ncof\nstroke\nmean pos\nTemp\nHumidity"
        n2645 = call <vilib>:"Query Available Printers.vi"() -> ("system configured printers"=w3469:string[])  [unwired: 9 in, 2 out]
        "System Configured Printers 2" <- w3469
        n2646 = local read "OK Button 16"() -> (w3466:bool)
        n2647 = Index Array(array=w3469, index="Select Printer 3") -> (element=w3471:string)
        "Selected Printer" <- w3471
        n2648 = case shown="True" "OK Button 16" {
          frame False {
          }
          frame True {
            n2649 = stacked-sequence {
              frame #0 {
                n2650 = local read "Numeric 16"() -> (w3794:i32)
                n2651 = local write "Numeric 10"(w3794) -> ()
              }
              frame #1 {
                n2652 = local read "S.NO"() -> (→"s.NO":string)
                n2653 = local read "String 29"() -> (w3798:string)
                n2654 = String To Path(string=w3798) -> (path=w3797:path)
                n2655 = Open/Create/Replace File "Open File"(file path (use dialog)=w3797) -> (refnum out=w3799:refnum<file>)  [unwired: 5 in, 2 out]
                n2656 = for {
                  N: 16 -> [_]
                  tunnel: w3799 -> [w3806]
                  i -> [w3802]
                  (unwired) TRUE ("line mode (F)")
                  n2657 = Read from Text File "Read File"(file (use dialog)=w3806) -> (text=w3800:string)  [unwired: 3 in, 3 out]
                  n2658 = Match Pattern(string=w3800, regular expression="(") -> (after substring=w3805:string)  [unwired: 1 in, 3 out]
                  n2659 = Match Pattern(string=w3805, regular expression=")") -> (before substring=w3801:string)  [unwired: 1 in, 3 out]
                  n2660 = case shown="1" w3802 {
                    tunnel: w3801 -> [w3807 w3808 _ _ w3809 w3810 w3811 w3813 w3815 w3817 w3819 w3821 w3823 w3825 _]
                    tunnel: w3800 -> [_ _ _ _ _ _ _ _ _ _ _ _ _ _ _]
                    frame 0 {
                      "TITTLE" <- w3807
                    }
                    frame 1 {
                      "Sample ID" <- w3808
                    }
                    frame 2 {
                    }
                    frame 3 {
                    }
                    frame 4 {
                      "Test Date" <- w3809
                    }
                    frame 5 {
                      "Tested by" <- w3810
                    }
                    frame 6 {
                      n2661 = Fract/Exp String To Number(string=w3811) -> (number=→"Humidity before test 2":dbl)  [unwired: 3 in, 1 out]
                    }
                    frame 7 {
                      n2662 = Fract/Exp String To Number(string=w3813) -> (number=→"Temperature before test 2":dbl)  [unwired: 3 in, 1 out]
                    }
                    frame 8 {
                      n2663 = Fract/Exp String To Number(string=w3815) -> (number=→"Humidity after test 2":dbl)  [unwired: 3 in, 1 out]
                    }
                    frame 9 {
                      n2664 = Fract/Exp String To Number(string=w3817) -> (number=→"Temperature after test 2":dbl)  [unwired: 3 in, 1 out]
                    }
                    frame 10 {
                      n2665 = Fract/Exp String To Number(string=w3819) -> (number=→"MWSD 2":dbl)  [unwired: 3 in, 1 out]
                    }
                    frame 11 {
                      n2666 = Fract/Exp String To Number(string=w3821) -> (number=→"AVP 2":dbl)  [unwired: 3 in, 1 out]
                    }
                    frame 12 {
                      n2667 = Fract/Exp String To Number(string=w3823) -> (number=→"HCF 2":dbl)  [unwired: 3 in, 1 out]
                    }
                    frame 13 {
                      n2668 = Fract/Exp String To Number(string=w3825) -> (number=→"WS1.4 2":dbl)  [unwired: 3 in, 1 out]
                    }
                    frame 14, Default {
                    }
                  }
                }
              }
              frame #2 {
              }
            }
            n2669 = local write "OK Button 16"(FALSE ("OK Button 13")) -> ()
          }
        }
        n2670 = disable-structure shown="Disabled" {
          frame Disabled {
            n2671 = case shown="True" "Export" {
              frame False {
              }
              frame True {
                w3477 = "                                      " ("string")
                w3479 = "\r"
                (unwired) i16 6 ("width (-)")
                w3556 = "\r"
                w3488 = "\r"
                n2672 = local write "Export"(FALSE ("Export")) -> ()
                n2673 = local read "String 29"() -> (w3525:string)
                n2674 = local read "String 39"() -> (w3495:string)
                n2675 = local read "String 38"() -> (w3498:string)
                n2676 = local read "String 37"() -> (w3504:string)
                n2677 = local read "String 36"() -> (w3501:string)
                n2678 = local read "String 35"() -> (w3508:string)
                n2679 = local read "String 34"() -> (w3513:string)
                n2680 = Match Pattern(string=w3525, regular expression=".dwm") -> (before substring=w3521:string)  [unwired: 1 in, 3 out]
                "before substring" <- w3521
                n2681 = local read "S 39"() -> (w3509:string)
                n2682 = local read "S 38"() -> (w3516:string)
                n2683 = local read "Temperature before test 2"() -> (w3545:dbl)
                n2684 = local read "Temperature after test 2"() -> (w3550:dbl)
                n2685 = local read "Humidity before test 2"() -> (w3531:dbl)
                n2686 = local read "Humidity after test 2"() -> (w3546:dbl)
                n2687 = local read "MWSD 2"() -> (w3542:dbl)
                n2688 = local read "WS1.4 2"() -> (w3558:dbl)
                n2689 = local read "HCF 2"() -> (w3554:dbl)
                n2690 = local read "AVP 2"() -> (w3543:dbl)
                n2691 = Concatenate Strings("8," ("string"), w3495) -> (w3496:string)
                n2692 = Concatenate Strings("7," ("string"), w3498) -> (w3499:string)
                n2693 = Concatenate Strings("6," ("string"), w3501) -> (w3502:string)
                n2694 = Concatenate Strings("5," ("string"), w3504) -> (w3505:string)
                n2695 = Concatenate Strings("4," ("string"), w3508) -> (w3507:string)
                n2696 = Concatenate Strings("3," ("string"), w3509) -> (w3511:string)
                n2697 = Concatenate Strings("2," ("string"), w3513) -> (w3512:string)
                n2698 = Concatenate Strings("1," ("string"), w3516) -> (w3515:string)
                n2699 = local read "Sample ID"() -> (w3563:string)
                n2700 = case shown="\"xlx\"" "Select File Type" {
                  tunnel: w3521 -> [w3566 w3568 w3570]
                  tunnel: [w3564 w3569 w3571] -> w3520
                  frame "xlx" {
                    n2701 = Concatenate Strings(w3566, ".xls" ("string")) -> (w3564:string)
                  }
                  frame "csv" {
                    n2702 = Concatenate Strings(w3568, ".csv" ("string")) -> (w3569:string)
                  }
                  frame "txt" {
                    n2703 = Concatenate Strings(w3570, ".txt" ("string")) -> (w3571:string)
                  }
                }
                n2704 = local read "Test Date"() -> (w3562:string)
                n2705 = local read "String 45"() -> (w3476:string)
                n2706 = local read "String 31"() -> (w3561:string)
                n2707 = local read "String 32"() -> (w3560:string)
                n2708 = local read "TITTLE"() -> (w3484:string)
                n2709 = Number To Fractional String(number=w3558, precision (6)=i16 2) -> (F-format string=w3559:string)  [unwired: 2 in]
                n2710 = Number To Fractional String(number=w3554, width (-)=i16 6, precision (6)=i16 2) -> (F-format string=w3555:string)  [unwired: 1 in]
                n2711 = Number To Fractional String(number=w3550, width (-)=i16 6, precision (6)=i16 2) -> (F-format string=w3549:string)  [unwired: 1 in]
                n2712 = Number To Fractional String(number=w3543, width (-)=i16 6, precision (6)=i16 2) -> (F-format string=w3541:string)  [unwired: 1 in]
                n2713 = Number To Fractional String(number=w3542, width (-)=i16 6, precision (6)=i16 2) -> (F-format string=w3540:string)  [unwired: 1 in]
                n2714 = Number To Fractional String(number=w3546, width (-)=i16 6, precision (6)=i16 2) -> (F-format string=w3544:string)  [unwired: 1 in]
                n2715 = Number To Fractional String(number=w3545, width (-)=i16 6, precision (6)=i16 2) -> (F-format string=w3551:string)  [unwired: 1 in]
                n2716 = Number To Fractional String(number=w3531, width (-)=i16 6, precision (6)=i16 2) -> (F-format string=w3530:string)  [unwired: 1 in]
                n2717 = local read "s.NO"() -> (w3478:string)
                n2718 = Concatenate Strings("=" ("string"), w3484) -> (w3483:string)
                n2719 = Concatenate Strings("S.No," ("string"), "                                       Parameters" ("string")) -> (w3489:string)
                n2720 = Concatenate Strings(w3556, w3515, w3530, w3556, w3512, w3551, w3556, w3511, w3544, w3556, w3507, w3549, w3556, w3505, w3540, w3556, w3502, w3541, w3556, w3499, w3555, w3556, w3496, w3559) -> (w3518:string)
                n2721 = Concatenate Strings(w3488, "," ("string"), w3476, w3478, w3477, w3560, w3563, w3477, w3561, w3562, w3488) -> (w3486:string)
                n2722 = local read "Tested by"() -> (w3492:string)
                n2723 = local read "String 33"() -> (w3493:string)
                n2724 = Concatenate Strings("," ("string"), "                                                                             " ("string")) -> (w3481:string)
                n2725 = Concatenate Strings(w3483, w3479, w3486, w3479, w3489, w3518, w3479, w3481, w3493, w3492) -> (→"export":string)
                n2726 = String To Path(string=w3520) -> (path=w3527:path)
